vi "Create AER.vi"(10 "Grid.lvclass":refnum<class "Grid.lvclass">, 11 "Synapses in":refnum<class "Synapses.lvclass">) -> (0 "No N":i32[](array[numeric]), 1 "W":dbl[](array[numeric]), 2 "PreIds":i32[](array[numeric]), 3 "AER.lvclass":refnum<class "AER.lvclass">)   [LabVIEW 2013, in "AER.lvclass"]
doc: "This VI creates the vectors for the AER implementation"
uses:
  AER.lvclass
  Synapses/Synapses.lvclass
  Controls/Type of Neuron.ctl
  Cube/Grid.lvclass
  Synapses/Synapses.lvclass/Synapses.ctl
  Cube/Grid.lvclass/Grid.ctl
  Neuron/Neuron.lvclass/Neuron.ctl
  AER.lvclass/AER.ctl
  Neuron/Get Neuron Properties.vi
panel:
  out "PFPC":i32[](array[numeric])
  in  "Neuron Type":T1
  out "NoPre":i32[](array[numeric])
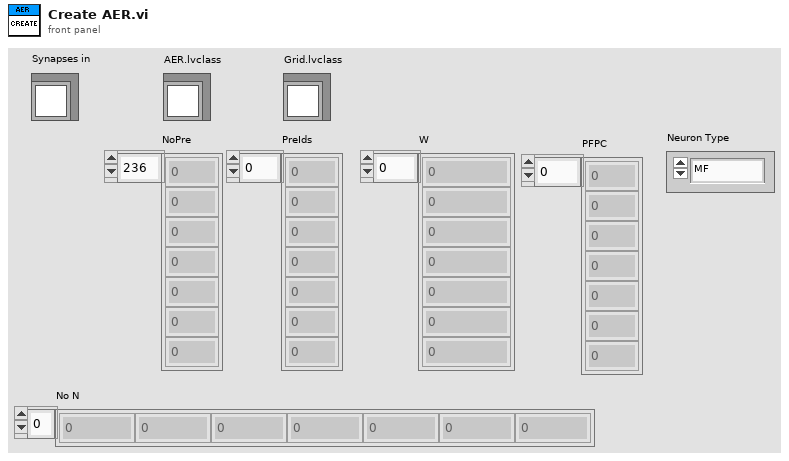
[diagram p1: front panel]
types:
  T1 = typedef "Type of Neuron.ctl" = enum16{"MF", "BA", "GO", "GC", "PC", "LU", "Glia (Dummy)"}
  T2 = typedef "Synapses.ctl" = cluster{"Synapse":T3, "Pre_List":i32[][], "Post_List":i32[][], "Weight gain":dbl}
  T3 = typedef "Type of Synapses.ctl" = enum16{"MF to GC", "GO to GC", "GC to GO", "MF to GO", "GC to PC", "GC to BA", "PC to BA", "BA to PC", "BA to GO"}
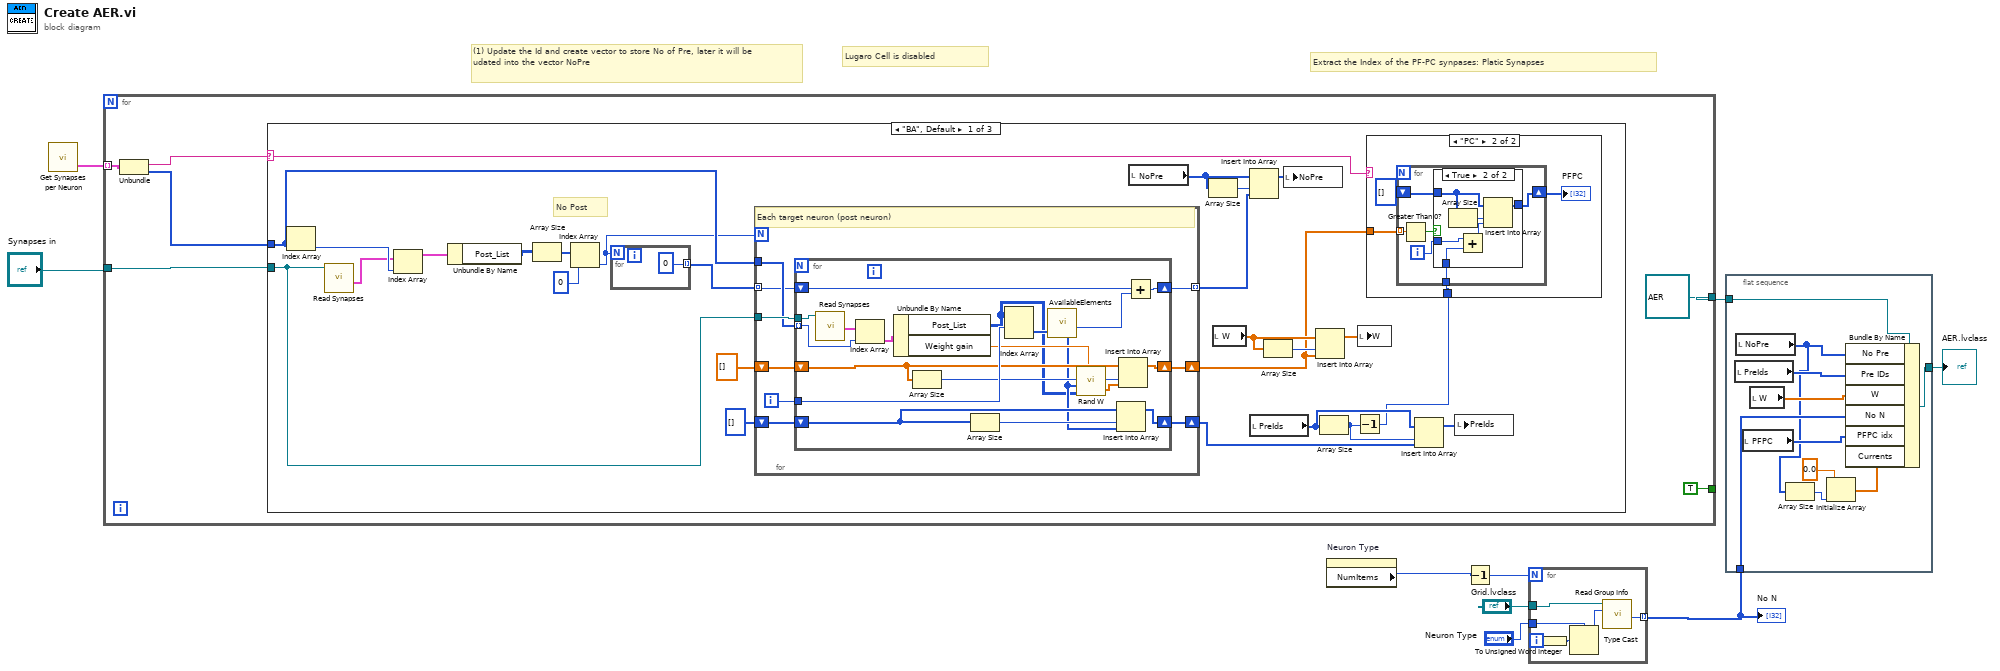
[diagram p0: block diagram]
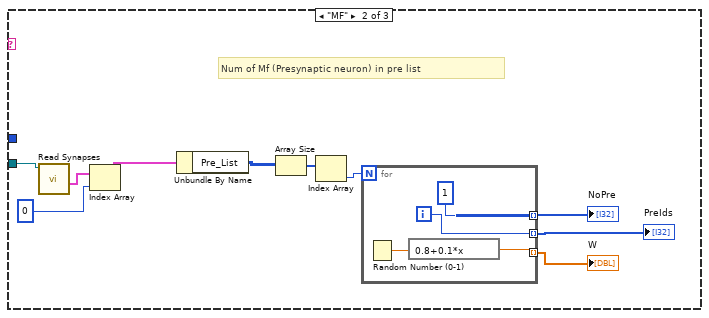
[diagram p4: hidden frame]
diagram:
  # "Lugaro Cell is disabled"
  # "Extract the Index of the PF-PC synpases: Platic Synapses"
  # "(1) Update the Id and create vector to store No of Pre, later it will be udated into the vector NoPre"
  n1 = call "Get Synapses per Neuron.vi"() -> ("Post Neurons Array"=w9:cluster{string, i32[]}[])  [unwired: 3 in]
  n2 = for {
    tunnel: w9 -> [w15] mode=indexing
    tunnel: "Synapses in" -> [w13]
    tunnel: [refnum<class "AER.lvclass"> refnum ("AER.lvclass")] -> w6
    tunnel: [TRUE] -> _
    n3 = Unbundle(w15) -> (w14:string, w10:i32[])
    n4 = case shown="\"BA\", Default" w14 {
      selector: w14 -> [w24 _ _]
      tunnel: w13 -> [w38 w91 _]
      tunnel: w10 -> [w39 _ _]
      frame "BA", Default {
        # "No Post"
        n5 = Index Array(array=w39) -> (element=w19:i32)  [unwired: 1 in]
        n6 = call "Read Synapses.vi"("Synapses in"=w38) -> ("Synapses"=w18:T2[])  [unwired: 7 in, 3 out]
        n7 = Index Array(array=w18, index=w19) -> (element=w20:T2)
        n8 = Unbundle By Name(w20) -> ("Post_List"=w40:i32[][])
        n9 = Array Size(array=w40) -> (size(s)=w41:i32[])
        n10 = Index Array(array=w41, index=0) -> (element=w17:i32)
        n11 = for {
          N: w17 -> [_]
          tunnel: [0] -> w37 mode=indexing
        }
        n12 = for {
          N: w17 -> [_]
          tunnel: w39 -> [w66]
          tunnel: w38 -> [w67]
          shift-right: [w61] -> w32
          shift-left: i32[] [] -> [w62]
          tunnel: w37 -> [w64] mode=indexing
          tunnel: [w63] -> w35 mode=indexing
          shift-right: [w59] -> w23
          shift-left: dbl[] [] -> [w60]
          i -> [w65]
          # "Each target neuron (post neuron)"
          n13 = for {
            tunnel: w67 -> [w86]
            tunnel: w66 -> [w69] mode=indexing
            tunnel: w65 -> [w85]
            shift-right: [w78] -> w61
            shift-left: w62 -> [w79]
            shift-right: [w83] -> w63
            shift-left: w64 -> [w82]
            shift-right: [w77] -> w59
            shift-left: w60 -> [w76]
            n14 = call "Read Synapses.vi"("Synapses in"=w86) -> ("Synapses"=w70:T2[])  [unwired: 7 in, 3 out]
            n15 = Index Array(array=w70, index=w69) -> (element=w68:T2)
            n16 = Unbundle By Name(w68) -> ("Post_List"=w71:i32[][], "Weight gain"=w73:dbl)
            n17 = Array Size(array=w76) -> (size(s)=w75:i32)
            n18 = Array Size(array=w79) -> (size(s)=w80:i32)
            n19 = Index Array(array=w71, index (row)=w85) -> (element=w81:i32[])  [unwired: 1 in]
            n20 = call "AvailableElements.vi"("Array"=w81) -> ("No Available"=w84:i32, "Occupied"=w72:i32[])  [unwired: 3 in]
            n21 = call "Rand W.vi"("Weight gain"=w73, "post"=w71, "Occupied"=w72) -> ("W Array"=w74:dbl[])  [unwired: 4 in]
            n22 = Insert Into Array(array=w79, index=w80, new element=w72) -> (w78:i32[])
            n23 = Insert Into Array(array=w76, index=w75, new element=w74) -> (w77:dbl[])
            n24 = Add(x=w82, y=w84) -> (x+y=w83:i32)
          }
        }
        n25 = local read "NoPre"() -> (w30:i32[])
        n26 = Array Size(array=w30) -> (size(s)=w29:i32)
        n27 = local read "W"() -> (w26:dbl[])
        n28 = Insert Into Array(array=w30, index=w29, new element=w35) -> (w36:i32[])
        n29 = local read "PreIds"() -> (w31:i32[])
        n30 = Array Size(array=w26) -> (size(s)=w27:i32)
        n31 = local write "NoPre"(w36) -> ()
        n32 = Insert Into Array(array=w26, index=w27, new element=w23) -> (w25:dbl[])
        n33 = Array Size(array=w31) -> (size(s)=w22:i32)
        n34 = Decrement(x=w22) -> (x-1=w21:i32)
        n35 = local write "W"(w25) -> ()
        n36 = case shown="\"PC\"" w24 {
          tunnel: w23 -> [_ w45]
          tunnel: w21 -> [_ w44]
          frame "False", Default {
          }
          frame "PC" {
            n37 = for {
              tunnel: w45 -> [w49] mode=indexing
              shift-right: [w51] -> w42
              shift-left: i32[] [] -> [w46]
              tunnel: w44 -> [w48]
              i -> [w47]
              n38 = Greater Than 0?(x=w49) -> (x > 0?=w50:bool)
              n39 = case shown="True" w50 {
                tunnel: [w52 w57] -> w51
                tunnel: w48 -> [_ w56]
                tunnel: w47 -> [_ w55]
                tunnel: w46 -> [w52 w53]
                frame False {
                }
                frame True {
                  n40 = Array Size(array=w53) -> (size(s)=w58:i32)
                  n41 = Add(x=w55, y=w56) -> (x+y=w54:i32)
                  n42 = Insert Into Array(array=w53, index=w58, new element=w54) -> (w57:i32[])
                }
              }
            }
            "PFPC" <- w42
          }
        }
        n43 = Insert Into Array(array=w31, index=w22, new element=w32) -> (w33:i32[])
        n44 = local write "PreIds"(w33) -> ()
      }
      frame "MF" {
        # "Num of Mf (Presynaptic neuron) in pre list"
        n45 = call "Read Synapses.vi"("Synapses in"=w91) -> ("Synapses"=w89:T2[])  [unwired: 7 in, 3 out]
        n46 = Index Array(array=w89, index=0 ("index synapses")) -> (element=w90:T2)
        n47 = Unbundle By Name(w90) -> ("Pre_List"=w97:i32[][])
        n48 = Array Size(array=w97) -> (size(s)=w96:i32[])
        n49 = Index Array(array=w96) -> (element=w95:i32)  [unwired: 1 in]
        n50 = for {
          N: w95 -> [_]
          tunnel: [1] -> w94 mode=indexing
          tunnel: [w98] -> w92 mode=indexing
          tunnel: [w100] -> w93 mode=indexing
          i -> [w100]
          n51 = Random Number (0-1)() -> (number: 0 to 1=w99:dbl)
          n52 = expression code="0.8+0.1*x"(w99) -> (w98:dbl)
        }
        "NoPre" <- w94
        "PreIds" <- w93
        "W" <- w92
      }
      frame "LU" {
        # "Lugaro Cell is disabled"
      }
    }
  }
  n53 = property on="Neuron Type" class="Enum (strict)"() -> ("NumItems"=w3:u32)  [unwired: 2 in, 2 out]
  n54 = Decrement(x=w3) -> (x-1=w2:u32)
  n55 = for {
    N: w2 -> [_]
    tunnel: "Grid.lvclass" -> [w107]
    tunnel: [w106] -> w1 mode=indexing
    tunnel: "Neuron Type" -> [w104]
    i -> [w103]
    n56 = To Unsigned Word Integer(number=w103) -> (unsigned 16bit integer=w102:u16)
    n57 = Type Cast(type=w104, x=w102) -> (*(type *) &x=w105:T1)
    n58 = call "Read Group Info.vi"("Neuron Type"=w105, "Grid in"=w107) -> ("N"=w106:i32)  [unwired: 7 in, 2 out]
  }
  "No N" <- w1
  n59 = flat-sequence {
    tunnel: [w117] -> w7
    tunnel: w6 -> [w116]
    tunnel: w1 -> [w114]
    frame #0 {
      n60 = local read "PreIds"() -> (w115:i32[])
      n61 = local read "NoPre"() -> (w108:i32[])
      n62 = local read "PFPC"() -> (w113:i32[])
      n63 = local read "W"() -> (w112:dbl[])
      n64 = Array Size(array=w108) -> (size(s)=w111:i32)
      n65 = Initialize Array(0.0 ("element"), w111) -> (w110:dbl[])
      n66 = Bundle By Name(cluster=w116, "No Pre"=w108, "Pre IDs"=w115, "W"=w112, "No N"=w114, "PFPC idx"=w113, "Currents"=w110) -> (w117:refnum<class "AER.lvclass">)
    }
  }
  "AER.lvclass" <- w7
